vi "Attenuator Abort Q Ops on Errors.vi"(8 "error in (no error)":errorcluster, 11 "Queue":refnum<queue>) -> (0 "error out":errorcluster)   [LabVIEW 2011]
uses:
  TypeDefs/Attenuator Queue Cluster.ctl
  TypeDefs/Attenuator Test Parameters.ctl
  TypeDefs/Attenuator Stimulus Parameters.ctl
  TypeDefs/Attenuator ATT Stimulus.ctl
  TypeDefs/Attenuator VNA Stimulus.ctl
  S Parameter/TypeDefs/SP Frequency Units.ctl
  TypeDefs/Attenuator VNA Calibration State.ctl
  TypeDefs/Attenuator Measurement Cluster.ctl
  TypeDefs/Attenuator Limit.ctl
  TypeDefs/Attenuator Calibration State.ctl
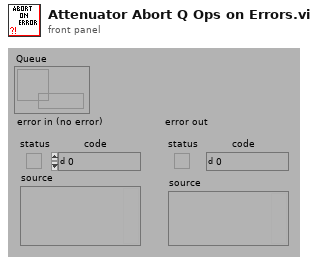
[diagram p1: front panel]
types:
  T1 = typedef "Attenuator Test Parameters.ctl" = cluster{"Stimulus":T2, "Measurement":T7, "Limit":T8, "Normalization":T9}
  T2 = typedef "Attenuator Stimulus Parameters.ctl" = cluster{"ATT Stimulus":T3, "VNA Stimulus":T4}
  T3 = typedef "Attenuator ATT Stimulus.ctl" = cluster{"Normalize":bool, "Value (dB)":dbl}
  T4 = typedef "Attenuator VNA Stimulus.ctl" = cluster{"Use Instrument Settings":bool, "Blank Frequencies":bool, "Sweep Type":enum32{"Linear", "Logarithmic", "List", "Power", "CW"}, "Sweep":cluster{"Fstart":dbl, "Fstop":dbl, "Units":T5, "Points":i32}, "Power (dBm)":dbl, "IFBW (Hz)":dbl, "Sweep Time (s)":dbl, "Calibration":T6}
  T5 = typedef "SP Frequency Units.ctl" = enum16{"Hz", "kHz", "MHz", "GHz", "Points"}
  T6 = typedef "Attenuator VNA Calibration State.ctl" = cluster{"State":bool, "String":string}
  T7 = typedef "Attenuator Measurement Cluster.ctl" = cluster{"Step (dB)":enum16{"0.25", "0.50", "1.00"}, "Start (dB)":dbl, "Stop (dB)":dbl}
  T8 = typedef "Attenuator Limit.ctl" = cluster{"Maximum Error":dbl}
  T9 = typedef "Attenuator Calibration State.ctl" = cluster{"Normalized?":bool, "Normalization Values (dB)":dbl[]}
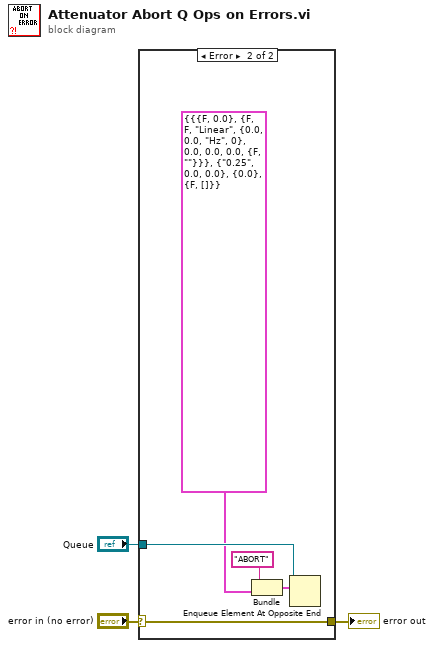
[diagram p0: block diagram]
diagram:
  n1 = case shown="Error" "error in (no error)" {
    selector: "error in (no error)" -> [w4 w8]
    tunnel: [w4 w8] -> w2
    tunnel: "Queue" -> [_ w6]
    frame No Error {
    }
    frame Error {
      n2 = Bundle("ABORT", "Test Parameters"=T1 {"Stimulus"={"ATT Stimulus"={"Normalize"=FALSE, "Value (dB)"=0.0}, "VNA Stimulus"={"Use Instrument Settings"=FALSE, "Blank Frequencies"=FALSE, "Sweep Type"=enum."Linear", "Sweep"={"Fstart"=0.0, "Fstop"=0.0, "Units"=enum."Hz", "Points"=0}, "Power (dBm)"=0.0, "IFBW (Hz)"=0.0, "Sweep Time (s)"=0.0, "Calibration"={"State"=FALSE, "String"=""}}}, "Measurement"={"Step (dB)"=enum."0.25", "Start (dB)"=0.0, "Stop (dB)"=0.0}, "Limit"={"Maximum Error"=0.0}, "Normalization"={"Normalized?"=FALSE, "Normalization Values (dB)"=[]}}) -> (w9:cluster{string, "Test Parameters":T1})  [unwired: 1 out]
      n3 = Enqueue Element At Opposite End(queue=w6, element=w9) -> ()  [unwired: 1 in, 4 out]
    }
  }
  "error out" <- w2
